vi "Concatenador_clusterSuper.vi"(0 "todos_os_dados_SAIDA(SPW)":T6, 5 "todos_os_dados_SAIDA(SPK)":T6, 7 "todos_os_dados_SAIDA(SKM)":T6, 9 "todos_os_dados_SAIDA(SKI)":T6, 11 "todos_os_dados_SAIDA(SKS)":T6) -> (8 "todos_os_dados_SAIDA(Final)":T6)   [LabVIEW 2019]
uses:
  \\SERVERPC\Server/padrao_todos_os_dados_SAIDA.ctl
  \\SERVERPC\Server/padrao_UCM.004.EEL.0300_SAIDA.ctl
  \\SERVERPC\Server/padrao_UCM.004.EEL.0200_SAIDA.ctl
  \\SERVERPC\Server/padrao_INTERNO.ctl
  \\SERVERPC\Server/padrao_ADAM_SAIDA.ctl
  \\SERVERPC\Server/padrao_array_variaveis_saida_SPW.ctl
  \\SERVERPC\Server/padrao_array_variaveis_saida_SPK.ctl
  \\SERVERPC\Server/padrao_array_variaveis_saida_SKI.ctl
  \\SERVERPC\Server/padrao_array_variaveis_saida_SKS.ctl
  \\SERVERPC\Server/padrao_array_variaveis_saida_SKM.ctl
panel:
  in  "Variaveis de saida SKM":T1=["AMS-EVC-001C", "AMS-EVC-001B", "AMS-ECV-001E", "AMS-FCV-005A", "AMS-FCV-004A", "WMS-FCV-001", "KMS-FCV-001", "ITN-SKMW-SI", "ITN-SKMK-SI", "ITN-SKMA-SI", "KMS-EVC-001", "AMS-EVC-001A", "WMS-EVC-001A", "WMS-EVC-001B", ""]
  in  "Variaveis de saida SKS":T2=["FSS-EVC-801", "FSS-EVC-802", "FSS-EVC-803", "CP-Y-601D", "CP-Y-601H", "FSS-EVC-804", "ITN-SS-SW-1", "ITN-SS-SK-1"]
  in  "Variaveis de saida SKI":T3=["FIS-EVC-031", "FIS-EVC-011", "FIS-EVC-012", "FIS-EVC-021", "FIS-EVC-022", "FIS-EVC-001", "FIS-EVC-002", "ITN-SI-SS-1", "ITN-SI-SS-2", "ITN-SI-SS-3"]
  in  "Variaveis de saida-SPK":T4=["KPS-EVC-001", "KPS-EVC-002", "KPS-EVC-003", "KPS-EVC-004", "KPS-EVC-005", "KPS-EVC-006", "KPS-EVC-007", "KPS-EVC-008", "KPS-WR-ON", "KPS-WR-OFF", "SPK-WR-VEL", "PID-KF-ON", "ITN-SPK-SKM", "KPS-FCV-001-W"]
  in  "Variaveis de saida-SPW":T5=["WPS-EVC-001", "WPS-EVC-002", "WPS-EVC-003", "WPS-EVC-004", "WPS-EVC-005", "WPS-EVC-006", "WPS-EVC-007", "WPS-EVC-008", "WPS-WR-ON", "WPS-WR-OFF", "SPW-WR-VEL", "PID-WF-ON", "ITN-SPW-SKM", "WPS-FCV-001-W"]
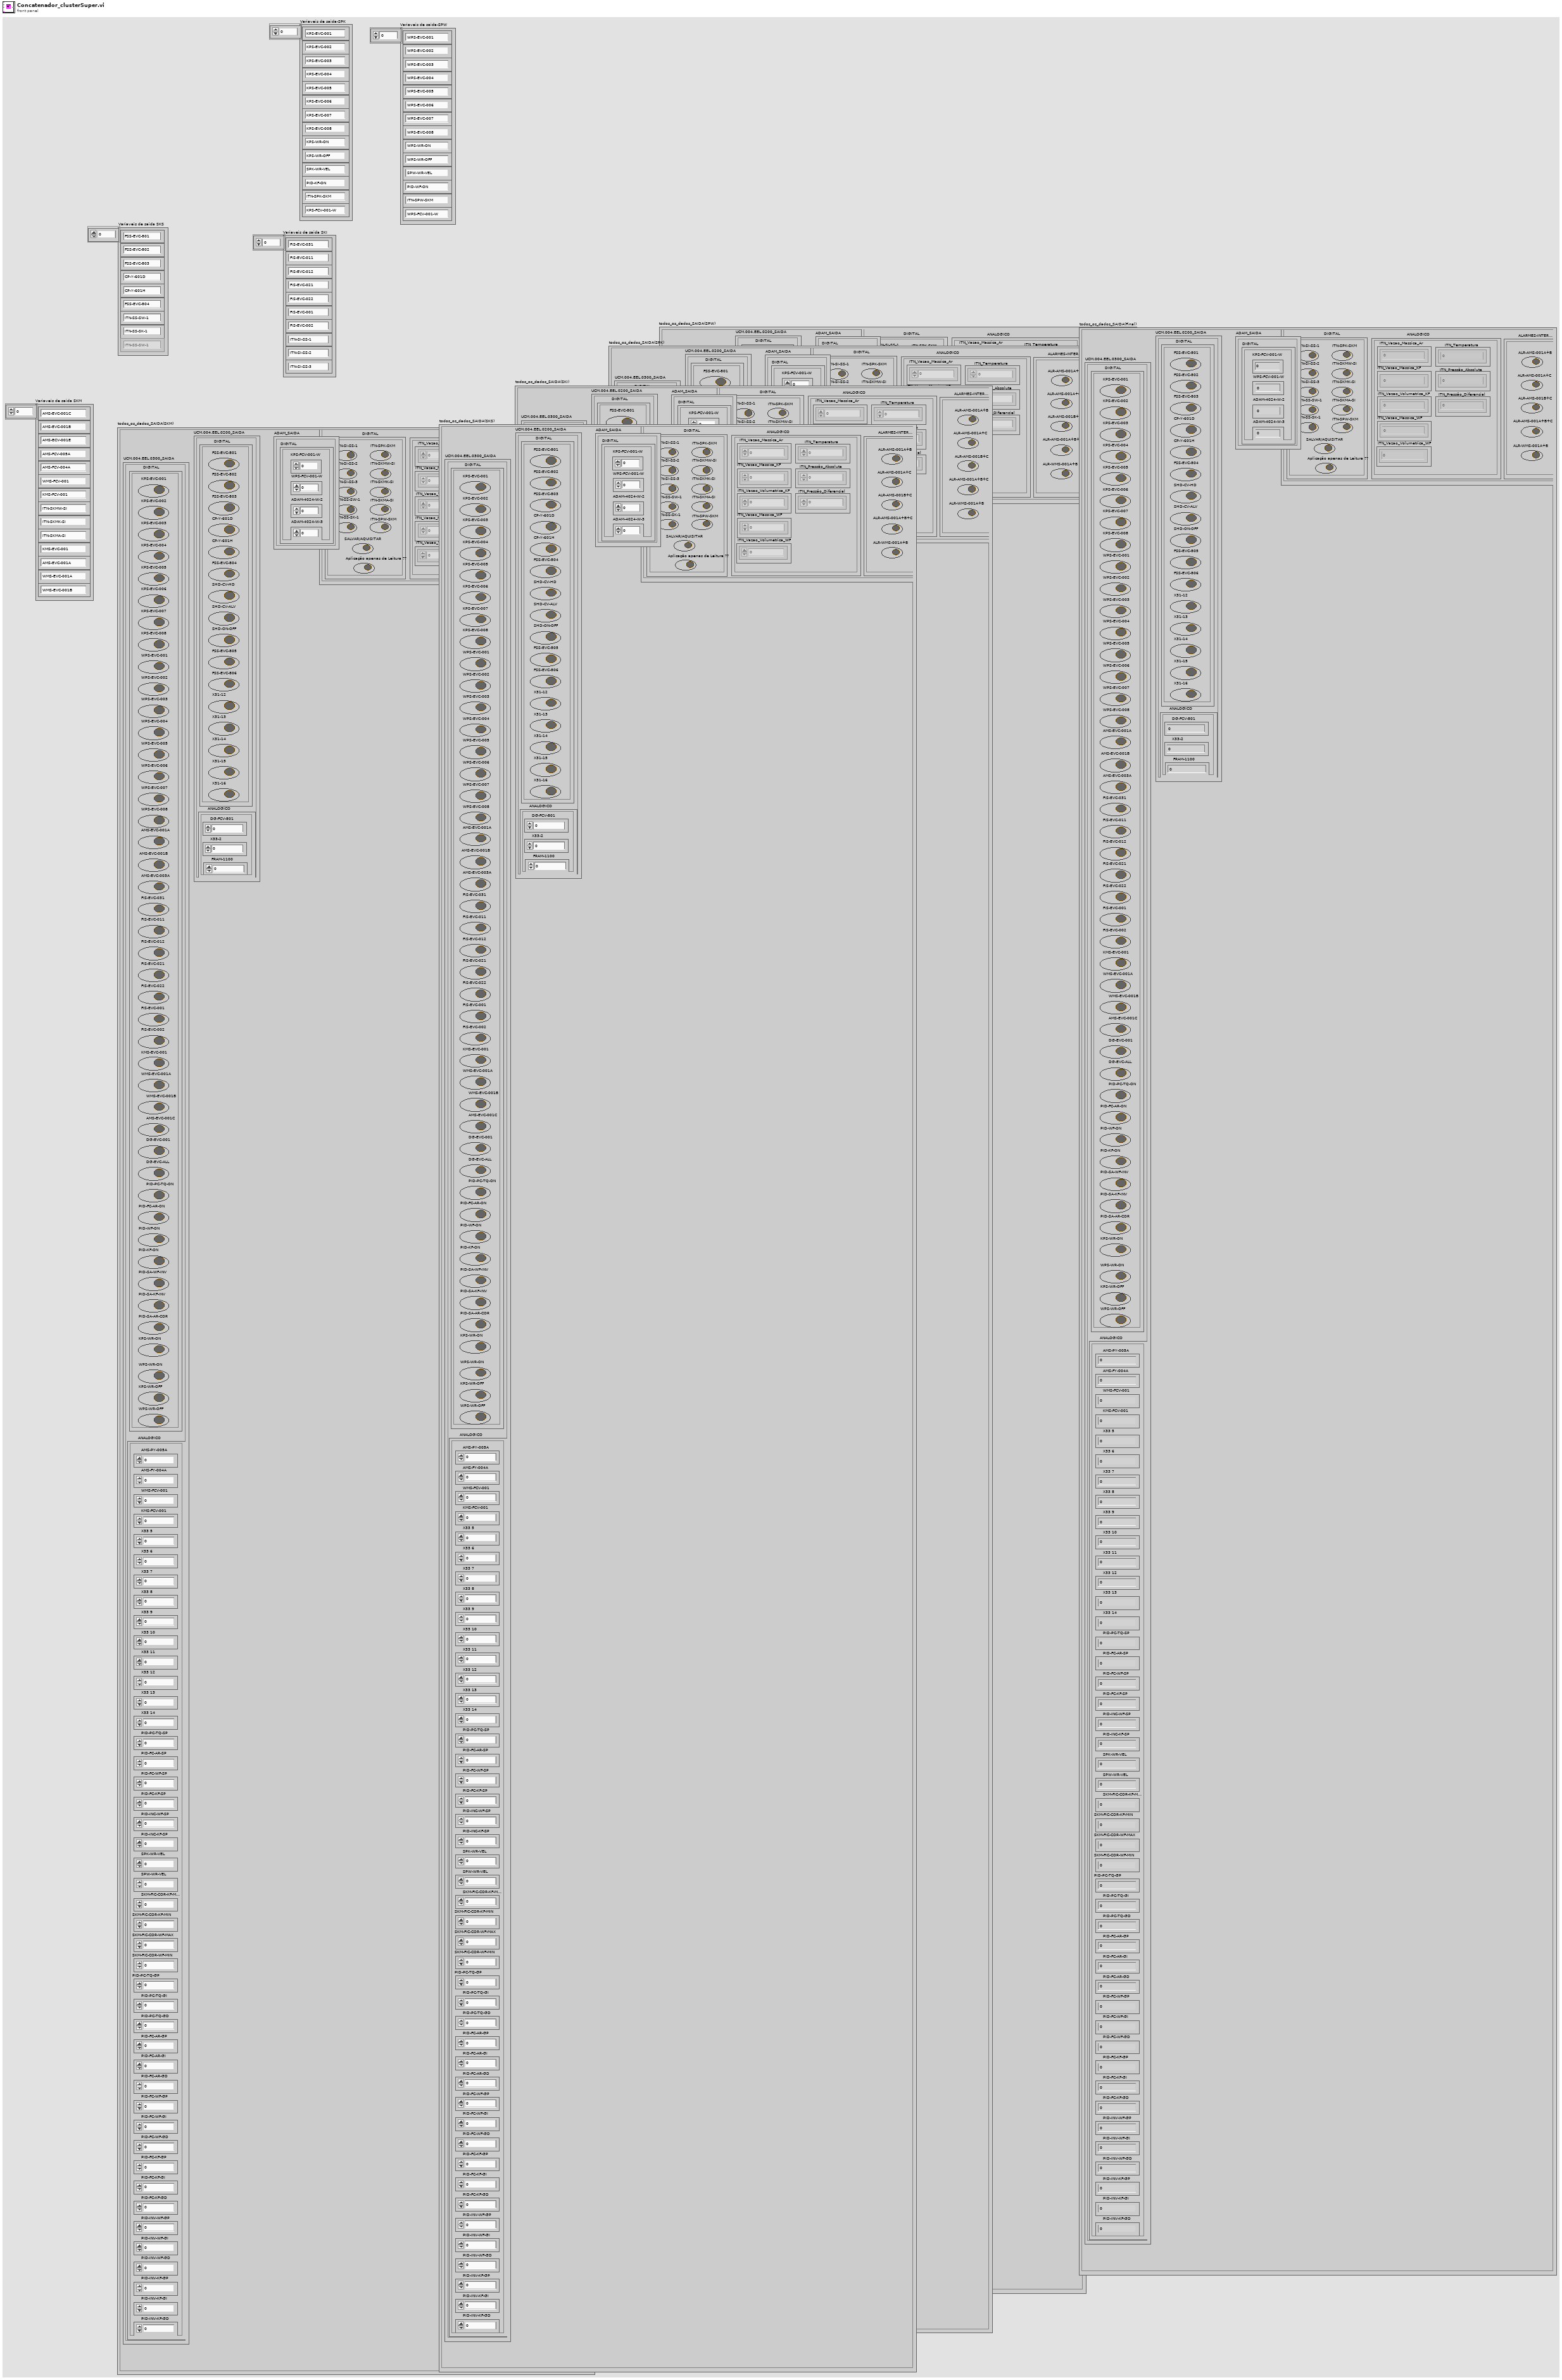
[diagram p1: front panel]
types:
  T1 = typedef "padrao_array_variaveis_saida_SKM.ctl" = string[]
  T2 = typedef "padrao_array_variaveis_saida_SKS.ctl" = string[]
  T3 = typedef "padrao_array_variaveis_saida_SKI.ctl" = string[]
  T4 = typedef "padrao_array_variaveis_saida_SPK.ctl" = string[]
  T5 = typedef "padrao_array_variaveis_saida_SPW.ctl" = string[]
  T6 = typedef "padrao_todos_os_dados_SAIDA.ctl" = cluster{"UCM.004.EEL.0300_SAIDA":T7, "UCM.004.EEL.0200_SAIDA":T8, "INTERNO":T9, "ADAM_SAIDA":T10}
  T7 = typedef "padrao_UCM.004.EEL.0300_SAIDA.ctl" = cluster{"DIGITAL":cluster{"KPS-EVC-001":bool, "KPS-EVC-002":bool, "KPS-EVC-003":bool, "KPS-EVC-004":bool, "KPS-EVC-005":bool, "KPS-EVC-006":bool, "KPS-EVC-007":bool, "KPS-EVC-008":bool, "WPS-EVC-001":bool, "WPS-EVC-002":bool, "WPS-EVC-003":bool, "WPS-EVC-004":bool, "WPS-EVC-005":bool, "WPS-EVC-006":bool, "WPS-EVC-007":bool, "WPS-EVC-008":bool, "AMS-EVC-001B":bool, "AMS-EVC-003A":bool, "FIS-EVC-031":bool, "FIS-EVC-011":bool, "FIS-EVC-012":bool, "FIS-EVC-021":bool, "FIS-EVC-022":bool, "FIS-EVC-001":bool, "FIS-EVC-002":bool, "KMS-EVC-001":bool, "WMS-EVC-001A":bool, "WMS-EVC-001B":bool, "AMS-EVC-001C":bool, "DG-EVC-001":bool, "DG-EVC-ALL":bool, "PID-PC-TQ-ON":bool, "PID-FC-AR-ON":bool, "PID-WF-ON":bool, "PID-KF-ON":bool, "PID-SA-WF-INV":bool, "PID-SA-KF-INV":bool, "PID-SA-AR-COR":bool, "KPS-WR-ON":bool, "WPS-WR-ON":bool, "KPS-WR-OFF":bool, "WPS-WR-OFF":bool, "AMS-EVC-001A":bool}, "ANALOGICO":cluster{"AMS-PY-005A":i16, "AMS-FY-004A":i16, "WMS-FCV-001":i16, "KMS-FCV-001":i16, "X33 5":i16, "X33 6":i16, "X33 7":i16, "X33 8":i16, "X33 9":i16, "X33 10":i16, "X33 11":i16, "X33 12":i16, "X33 13":i16, "X33 14":i16, "PID-PC-TQ-SP":i16, "PID-FC-AR-SP":i16, "PID-FC-WF-SP":i16, "PID-FC-KF-SP":i16, "PID-INC-WF-SP":i16, "PID-INC-KF-SP":i16, "SPK-WR-VEL":i32, "SPW-WR-VEL":i32, "SKM-FIC-COR-KF-MAX":dbl, "SKM-FIC-COR-KF-MIN":dbl, "SKM-FIC-COR-WF-MAX":dbl, "SKM-FIC-COR-WF-MIN":dbl, "PID-PC-TQ-GP":dbl, "PID-PC-TQ-GI":dbl, "PID-PC-TQ-GD":dbl, "PID-FC-AR-GP":dbl, "PID-FC-AR-GI":dbl, "PID-FC-AR-GD":dbl, "PID-FC-WF-GP":dbl, "PID-FC-WF-GI":dbl, "PID-FC-WF-GD":dbl, "PID-FC-KF-GP":dbl, "PID-FC-KF-GI":dbl, "PID-FC-KF-GD":dbl, "PID-INV-WF-GP":dbl, "PID-INV-WF-GI":dbl, "PID-INV-WF-GD":dbl, "PID-INV-KF-GP":dbl, "PID-INV-KF-GI":dbl, "PID-INV-KF-GD":dbl}}
  T8 = typedef "padrao_UCM.004.EEL.0200_SAIDA.ctl" = cluster{"DIGITAL":cluster{"FSS-EVC-801":bool, "FSS-EVC-802":bool, "FSS-EVC-803":bool, "CP-Y-601D":bool, "CP-Y-601H":bool, "FSS-EVC-804":bool, "SHD-CV-HD":bool, "SHD-CV-ALV":bool, "SHD-ON-OFF":bool, "FSS-EVC-805":bool, "FSS-EVC-806":bool, "X31-12":bool, "X31-13":bool, "X31-14":bool, "X31-15":bool, "X31-16":bool}, "ANALOGICO":cluster{"DG-FCV-801":i16, "X33-2":i16, "FRAM-1100":i16}}
  T9 = typedef "padrao_INTERNO.ctl" = cluster{"DIGITAL":cluster{"ITN-SI-SS-1":bool, "ITN-SI-SS-2":bool, "ITN-SI-SS-3":bool, "ITN-SS-SW-1":bool, "ITN-SS-SK-1":bool, "ITN-SPW-SKM":bool, "ITN-SKMW-SI":bool, "ITN-SKMK-SI":bool, "ITN-SKMA-SI":bool, "ITN-SPK-SKM":bool, "Aplicação apenas de Leitura ??":bool, "SALVAR/AQUISITAR":bool}, "ANALOGICO":cluster{"ITN_Vazao_Massica_Ar":dbl[], "ITN_Vazao_Volumetrica_WF":dbl[], "ITN_Vazao_Massica_KF":dbl[], "ITN_Vazao_Massica_WF":dbl[], "ITN_Vazao_Volumetrica_KF":dbl[], "ITN_Temperatura":dbl[], "ITN_Pressão_Absoluta":dbl[], "ITN_Pressão_Diferencial":dbl[]}, "ALARMES-INTERNOS":cluster{"ALR-AMS-001A+B":bool, "ALR-AMS-001A+C":bool, "ALR-AMS-001B+C":bool, "ALR-AMS-001A+B+C":bool, "ALR-WMS-001A+B":bool}}
  T10 = typedef "padrao_ADAM_SAIDA.ctl" = cluster{"DIGITAL":cluster{"KPS-FCV-001-W":dbl, "WPS-FCV-001-W":dbl, "ADAM-4024-W-2":dbl, "ADAM-4024-W-3":dbl}}
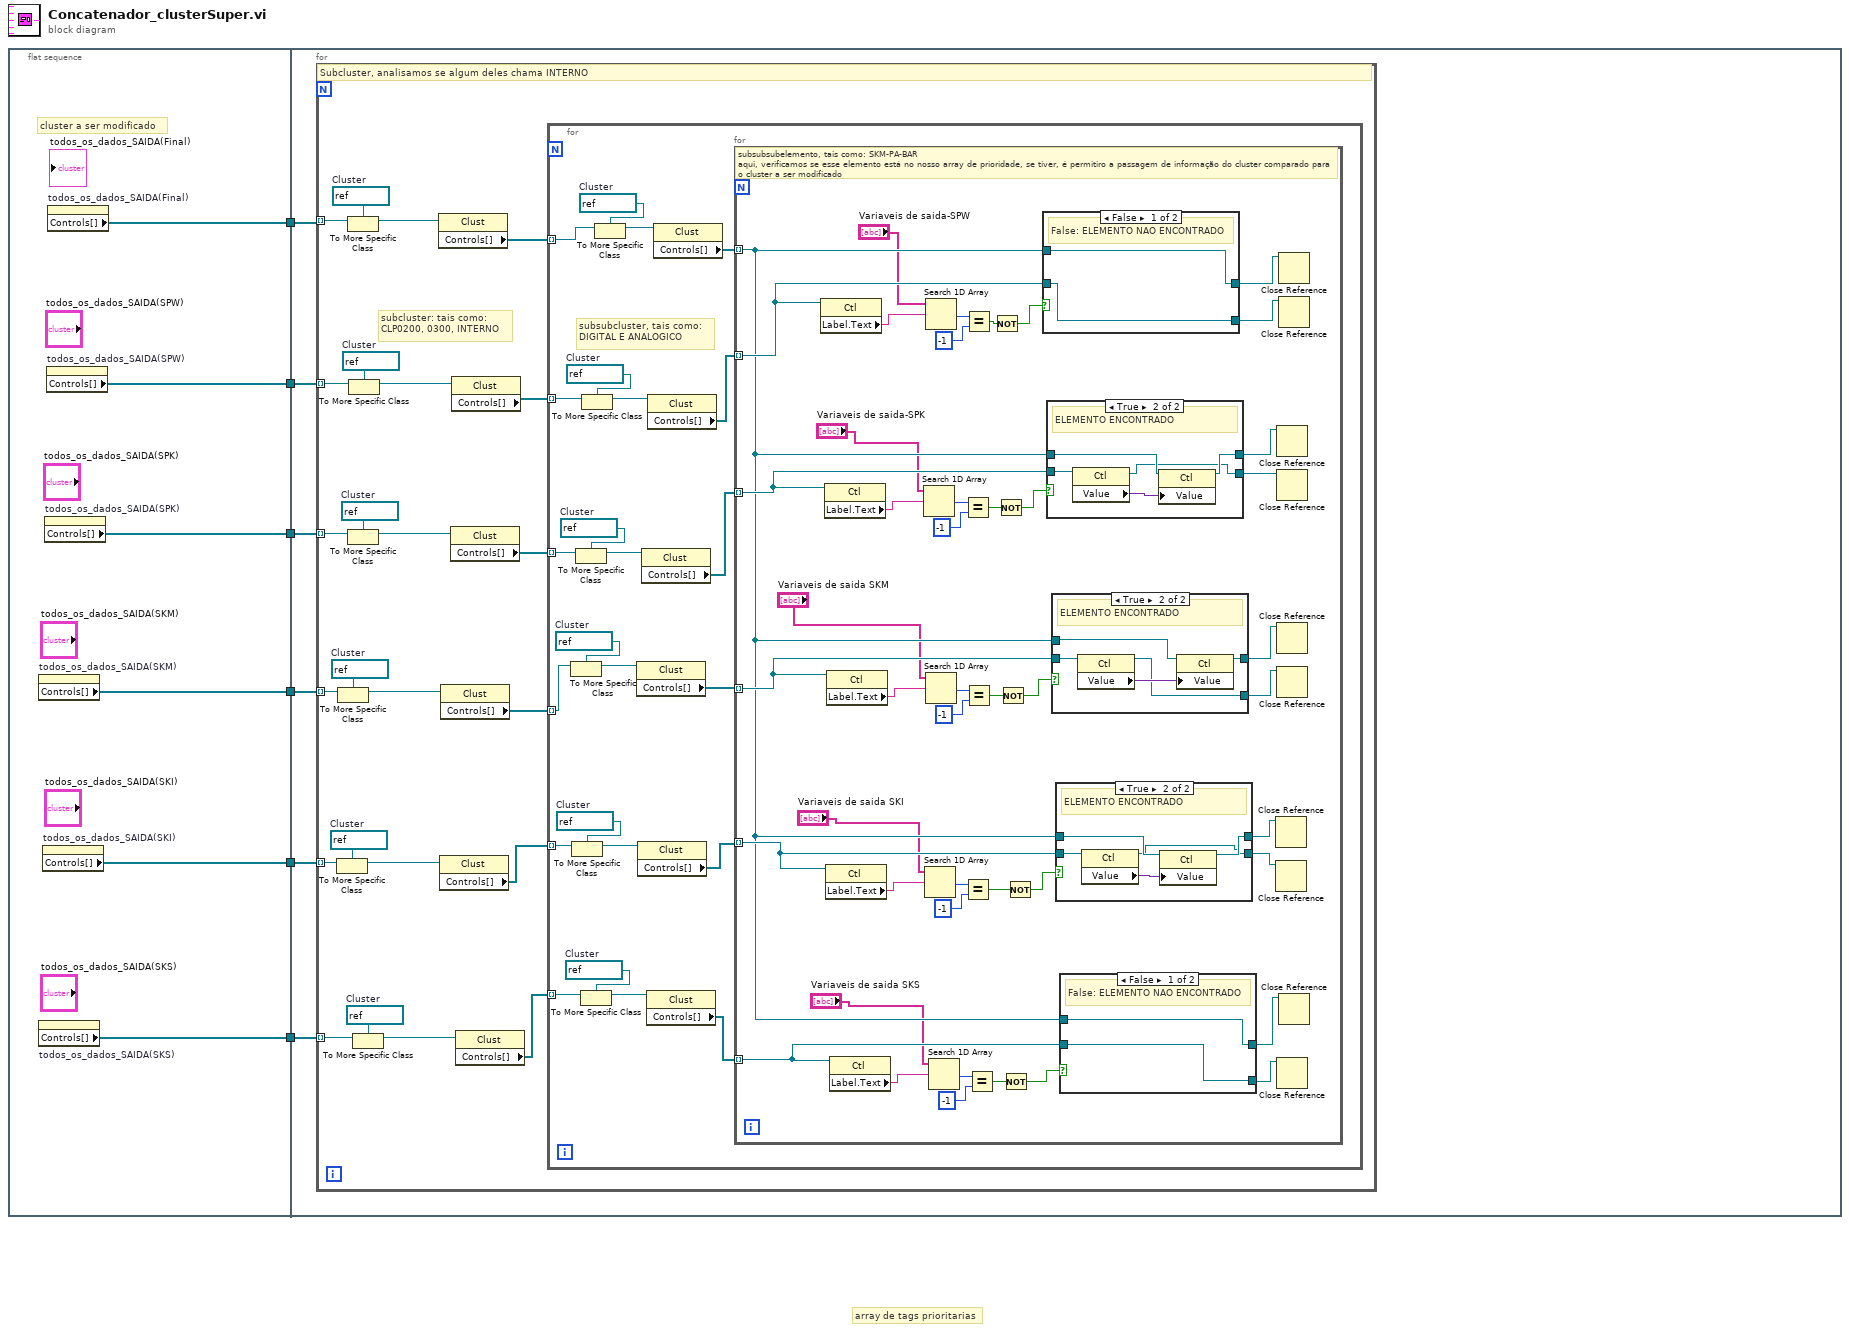
[diagram p0: block diagram]
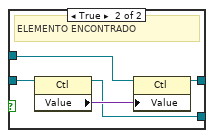
[diagram p2: hidden frame]
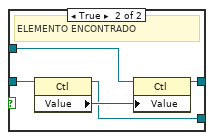
[diagram p6: hidden frame]
diagram:
  # "array de tags prioritarias"
  n1 = flat-sequence {
    tunnel: [w10] -> w6
    tunnel: [w12] -> w5
    tunnel: [w11] -> w4
    tunnel: [w9] -> w3
    tunnel: [w8] -> w2
    tunnel: [w7] -> w1
    tunnel: w6 -> [w18]
    tunnel: w5 -> [w17]
    tunnel: w4 -> [w16]
    tunnel: w3 -> [w15]
    tunnel: w2 -> [w14]
    tunnel: w1 -> [w13]
    frame #0 {
      # "cluster a ser modificado"
      # "Nessa parte, entra o array de cluster, há um filtro que devolve apenas um array de string\ncom as tags interessantes.\né criada uma referencia do cluster que sera comparado e abre a referencia do cluster a ser modificado"
      n2 = property on="todos_os_dados_SAIDA(SKM)" class="Clust (strict)"() -> ("Controls[]"=w9:refnum<vi>[])  [unwired: 2 in, 2 out]
      n3 = property on="todos_os_dados_SAIDA(SKS)" class="Clust (strict)"() -> ("Controls[]"=w7:refnum<vi>[])  [unwired: 2 in, 2 out]
      n4 = property on="todos_os_dados_SAIDA(SKI)" class="Clust (strict)"() -> ("Controls[]"=w8:refnum<vi>[])  [unwired: 2 in, 2 out]
      n5 = property on="todos_os_dados_SAIDA(SPK)" class="Clust (strict)"() -> ("Controls[]"=w11:refnum<vi>[])  [unwired: 2 in, 2 out]
      n6 = property on="todos_os_dados_SAIDA(SPW)" class="Clust (strict)"() -> ("Controls[]"=w12:refnum<vi>[])  [unwired: 2 in, 2 out]
      n7 = property on="todos_os_dados_SAIDA(Final)" class="Clust (strict)"() -> ("Controls[]"=w10:refnum<vi>[])  [unwired: 2 in, 2 out]
    }
    frame #1 {
      # "O primeiro loop entra dentro dos sub cluster do cluster global, caso eles forem INTERNO, não itera sobre ele , pois nao existe prioridade no cluster INTERNO.\nDentro do subsubcluster, novamente iteramos para acessarmos os subsubcluster existentes, tais como DIGITAL e ANALOGICO.\nDentro dos subsubsubcluster, iteramos para achar cada variavel, verificamos se essa variavel pertence ao grupo dos prioritarios (array de prioridade), e se sim, a informação é passado do cluster de todos os dados comparado para o cluster de todos os dados a ser modificado"
      n8 = for {
        tunnel: w18 -> [w39] mode=indexing
        tunnel: w17 -> [w35] mode=indexing
        tunnel: w16 -> [w32] mode=indexing
        tunnel: w15 -> [w24] mode=indexing
        tunnel: w14 -> [w23] mode=indexing
        tunnel: w13 -> [w19] mode=indexing
        w21 = refnum<vi> refnum  # Cluster
        w29 = refnum<vi> refnum  # Cluster
        w25 = refnum<vi> refnum  # Cluster
        w33 = refnum<vi> refnum  # Cluster
        w38 = refnum<vi> refnum  # Cluster
        w42 = refnum<vi> refnum  # Cluster
        # "subcluster: tais como:\nCLP0200, 0300, INTERNO"
        # "Subcluster, analisamos se algum deles chama INTERNO"
        n9 = To More Specific Class(target class=w29, reference=w23) -> (specific class reference=w28:refnum<vi>)  [unwired: 1 in, 1 out]
        n10 = To More Specific Class(target class=w25, reference=w24) -> (specific class reference=w27:refnum<vi>)  [unwired: 1 in, 1 out]
        n11 = To More Specific Class(target class=w42, reference=w39) -> (specific class reference=w40:refnum<vi>)  [unwired: 1 in, 1 out]
        n12 = To More Specific Class(target class=w33, reference=w32) -> (specific class reference=w34:refnum<vi>)  [unwired: 1 in, 1 out]
        n13 = To More Specific Class(target class=w38, reference=w35) -> (specific class reference=w36:refnum<vi>)  [unwired: 1 in, 1 out]
        n14 = To More Specific Class(target class=w21, reference=w19) -> (specific class reference=w22:refnum<vi>)  [unwired: 1 in, 1 out]
        n15 = property on="Property Node" class="Clust"(reference=w40) -> ("Controls[]"=w41:refnum<vi>[])  [unwired: 1 in, 2 out]
        n16 = property on="Property Node" class="Clust"(reference=w28) -> ("Controls[]"=w30:refnum<vi>[])  [unwired: 1 in, 2 out]
        n17 = property on="Property Node" class="Clust"(reference=w27) -> ("Controls[]"=w26:refnum<vi>[])  [unwired: 1 in, 2 out]
        n18 = property on="Property Node" class="Clust"(reference=w34) -> ("Controls[]"=w31:refnum<vi>[])  [unwired: 1 in, 2 out]
        n19 = property on="Property Node" class="Clust"(reference=w36) -> ("Controls[]"=w37:refnum<vi>[])  [unwired: 1 in, 2 out]
        n20 = property on="Property Node" class="Clust"(reference=w22) -> ("Controls[]"=w20:refnum<vi>[])  [unwired: 1 in, 2 out]
        n21 = for {
          tunnel: w41 -> [w65] mode=indexing
          tunnel: w37 -> [w60] mode=indexing
          tunnel: w31 -> [w56] mode=indexing
          tunnel: w26 -> [w51] mode=indexing
          tunnel: w30 -> [w54] mode=indexing
          tunnel: w20 -> [w44] mode=indexing
          w45 = refnum<vi> refnum  # Cluster
          w53 = refnum<vi> refnum  # Cluster
          w49 = refnum<vi> refnum  # Cluster
          w57 = refnum<vi> refnum  # Cluster
          w62 = refnum<vi> refnum  # Cluster
          w64 = refnum<vi> refnum  # Cluster
          # "subsubcluster, tais como:\nDIGITAL E ANALOGICO"
          n22 = To More Specific Class(target class=w49, reference=w51) -> (specific class reference=w50:refnum<vi>)  [unwired: 1 in, 1 out]
          n23 = To More Specific Class(target class=w53, reference=w54) -> (specific class reference=w52:refnum<vi>)  [unwired: 1 in, 1 out]
          n24 = To More Specific Class(target class=w57, reference=w56) -> (specific class reference=w58:refnum<vi>)  [unwired: 1 in, 1 out]
          n25 = To More Specific Class(target class=w45, reference=w44) -> (specific class reference=w46:refnum<vi>)  [unwired: 1 in, 1 out]
          n26 = To More Specific Class(target class=w62, reference=w60) -> (specific class reference=w61:refnum<vi>)  [unwired: 1 in, 1 out]
          n27 = To More Specific Class(target class=w64, reference=w65) -> (specific class reference=w66:refnum<vi>)  [unwired: 1 in, 1 out]
          n28 = property on="Property Node" class="Clust"(reference=w50) -> ("Controls[]"=w48:refnum<vi>[])  [unwired: 1 in, 2 out]
          n29 = property on="Property Node" class="Clust"(reference=w52) -> ("Controls[]"=w47:refnum<vi>[])  [unwired: 1 in, 2 out]
          n30 = property on="Property Node" class="Clust"(reference=w58) -> ("Controls[]"=w55:refnum<vi>[])  [unwired: 1 in, 2 out]
          n31 = property on="Property Node" class="Clust"(reference=w46) -> ("Controls[]"=w43:refnum<vi>[])  [unwired: 1 in, 2 out]
          n32 = property on="Property Node" class="Clust"(reference=w61) -> ("Controls[]"=w59:refnum<vi>[])  [unwired: 1 in, 2 out]
          n33 = property on="Property Node" class="Clust"(reference=w66) -> ("Controls[]"=w63:refnum<vi>[])  [unwired: 1 in, 2 out]
          n34 = for {
            tunnel: w63 -> [w82] mode=indexing
            tunnel: w59 -> [w108] mode=indexing
            tunnel: w55 -> [w101] mode=indexing
            tunnel: w48 -> [w90] mode=indexing
            tunnel: w47 -> [w89] mode=indexing
            tunnel: w43 -> [w83] mode=indexing
            # "subsubsubelemento, tais como: SKM-PA-BAR\naqui, verificamos se esse elemento está no nosso array de prioridade, se tiver, é permitiro a passagem de informação do cluster comparado para o cluster a ser modificado"
            n35 = property class="Ctl"(reference=w108) -> ("Label.Text"=w107:string)  [unwired: 1 in, 2 out]
            n36 = property class="Ctl"(reference=w101) -> ("Label.Text"=w106:string)  [unwired: 1 in, 2 out]
            n37 = property class="Ctl"(reference=w89) -> ("Label.Text"=w96:string)  [unwired: 1 in, 2 out]
            n38 = property class="Ctl"(reference=w90) -> ("Label.Text"=w95:string)  [unwired: 1 in, 2 out]
            n39 = property class="Ctl"(reference=w83) -> ("Label.Text"=w88:string)  [unwired: 1 in, 2 out]
            n40 = Search 1D Array(1D array="Variaveis de saida-SPK", element=w106) -> (index of element=w102:i32)  [unwired: 1 in]
            n41 = Search 1D Array(1D array="Variaveis de saida SKI", element=w96) -> (index of element=w100:i32)  [unwired: 1 in]
            n42 = Search 1D Array(1D array="Variaveis de saida-SPW", element=w107) -> (index of element=w112:i32)  [unwired: 1 in]
            n43 = Search 1D Array(1D array="Variaveis de saida SKM", element=w95) -> (index of element=w91:i32)  [unwired: 1 in]
            n44 = Search 1D Array(1D array="Variaveis de saida SKS", element=w88) -> (index of element=w84:i32)  [unwired: 1 in]
            n45 = Equal?(x=w102, y=-1) -> (x = y?=w104:bool)
            n46 = Equal?(x=w100, y=-1) -> (x = y?=w98:bool)
            n47 = Equal?(x=w112, y=-1) -> (x = y?=w110:bool)
            n48 = Equal?(x=w91, y=-1) -> (x = y?=w93:bool)
            n49 = Equal?(x=w84, y=-1) -> (x = y?=w86:bool)
            n50 = Not(x=w110) -> (.not. x?=w109:bool)
            n51 = Not(x=w104) -> (.not. x?=w105:bool)
            n52 = Not(x=w93) -> (.not. x?=w94:bool)
            n53 = Not(x=w86) -> (.not. x?=w87:bool)
            n54 = Not(x=w98) -> (.not. x?=w97:bool)
            n55 = case shown="False" w109 {
              tunnel: w82 -> [w142 w147]
              tunnel: w108 -> [w141 w146]
              tunnel: [w142 w144] -> w81
              tunnel: [w141 w143] -> w80
              frame False {
                # "False: ELEMENTO NAO ENCONTRADO"
              }
              frame True {
                # "ELEMENTO ENCONTRADO"
                n56 = property class="Ctl"(reference=w146) -> (reference out=w143:refnum<vi>, "Value"=w145:variant)  [unwired: 1 in, 1 out]
                n57 = property class="Ctl"(reference=w147, "Value"=w145) -> (reference out=w144:refnum<vi>)  [unwired: 1 in, 1 out]
              }
            }
            n58 = case shown="True" w105 {
              tunnel: w82 -> [w135 w139]
              tunnel: w101 -> [w134 w138]
              tunnel: [w135 w137] -> w79
              tunnel: [w134 w136] -> w78
              frame False {
                # "False: ELEMENTO NAO ENCONTRADO"
              }
              frame True {
                # "ELEMENTO ENCONTRADO"
                n59 = property class="Ctl"(reference=w138) -> (reference out=w136:refnum<vi>, "Value"=w140:variant)  [unwired: 1 in, 1 out]
                n60 = property class="Ctl"(reference=w139, "Value"=w140) -> (reference out=w137:refnum<vi>)  [unwired: 1 in, 1 out]
              }
            }
            n61 = case shown="True" w94 {
              tunnel: w82 -> [w128 w133]
              tunnel: w90 -> [w127 w132]
              tunnel: [w128 w130] -> w77
              tunnel: [w127 w129] -> w76
              frame False {
                # "False: ELEMENTO NAO ENCONTRADO"
              }
              frame True {
                # "ELEMENTO ENCONTRADO"
                n62 = property class="Ctl"(reference=w132) -> (reference out=w129:refnum<vi>, "Value"=w131:variant)  [unwired: 1 in, 1 out]
                n63 = property class="Ctl"(reference=w133, "Value"=w131) -> (reference out=w130:refnum<vi>)  [unwired: 1 in, 1 out]
              }
            }
            n64 = case shown="True" w97 {
              tunnel: w82 -> [w121 w125]
              tunnel: w89 -> [w120 w124]
              tunnel: [w121 w123] -> w75
              tunnel: [w120 w122] -> w74
              frame False {
                # "False: ELEMENTO NAO ENCONTRADO"
              }
              frame True {
                # "ELEMENTO ENCONTRADO"
                n65 = property class="Ctl"(reference=w124) -> (reference out=w122:refnum<vi>, "Value"=w126:variant)  [unwired: 1 in, 1 out]
                n66 = property class="Ctl"(reference=w125, "Value"=w126) -> (reference out=w123:refnum<vi>)  [unwired: 1 in, 1 out]
              }
            }
            n67 = case shown="False" w87 {
              tunnel: w83 -> [w113 w118]
              tunnel: w82 -> [w114 w117]
              tunnel: [w114 w116] -> w73
              tunnel: [w113 w115] -> w72
              frame False {
                # "False: ELEMENTO NAO ENCONTRADO"
              }
              frame True {
                # "ELEMENTO ENCONTRADO"
                n68 = property class="Ctl"(reference=w118) -> (reference out=w115:refnum<vi>, "Value"=w119:variant)  [unwired: 1 in, 1 out]
                n69 = property class="Ctl"(reference=w117, "Value"=w119) -> (reference out=w116:refnum<vi>)  [unwired: 1 in, 1 out]
              }
            }
            n70 = Close Reference(reference=w75) -> ()  [unwired: 1 in, 1 out]
            n71 = Close Reference(reference=w74) -> ()  [unwired: 1 in, 1 out]
            n72 = Close Reference(reference=w79) -> ()  [unwired: 1 in, 1 out]
            n73 = Close Reference(reference=w78) -> ()  [unwired: 1 in, 1 out]
            n74 = Close Reference(reference=w77) -> ()  [unwired: 1 in, 1 out]
            n75 = Close Reference(reference=w76) -> ()  [unwired: 1 in, 1 out]
            n76 = Close Reference(reference=w72) -> ()  [unwired: 1 in, 1 out]
            n77 = Close Reference(reference=w81) -> ()  [unwired: 1 in, 1 out]
            n78 = Close Reference(reference=w80) -> ()  [unwired: 1 in, 1 out]
            n79 = Close Reference(reference=w73) -> ()  [unwired: 1 in, 1 out]
          }
        }
      }
    }
  }
